vi "Memory.Truncate I64 to I32.vi"(11 "I64":i64) -> (3 "truncated I32":i32)   [LabVIEW 2016, in "LabVIEW Memory Manager.lvlib"]
uses:
  LabVIEW Memory Manager.lvlib
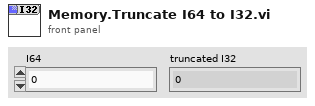
[diagram p1: front panel]
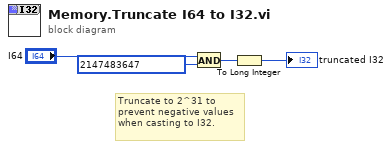
[diagram p0: block diagram]
diagram:
  # "Truncate to 2^31 to prevent negative values when casting to I32."
  n1 = And(x="I64", y=i64 2147483647) -> (x .and. y?=w2:i64)
  n2 = To Long Integer(number=w2) -> (32bit integer=→"truncated I32":i32)
